vi "Nattify - Arrange FP Controls Rows.vi"(0 "sorted array of control info":T2[](array[typedef]), 1 "FP objects arrangement info":T1, 11 "error in":errorcluster) -> (15 "error out":errorcluster)   [LabVIEW 2020]
uses:
  Nattify - FP Control Info.ctl
  <vilib>/Utility/miscctls.llb/LVRectTypeDef.ctl
  Nattify - FP Objects Arrangement Info.ctl
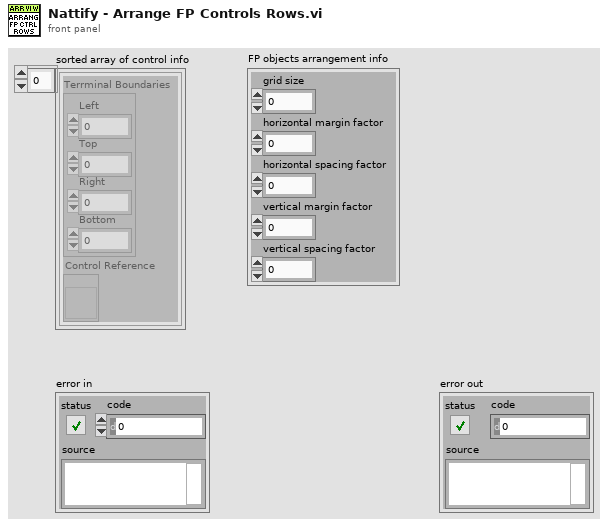
[diagram p1: front panel]
types:
  T1 = typedef "Nattify - FP Objects Arrangement Info.ctl" = cluster{"grid size":i32, "horizontal margin factor":i32, "horizontal spacing factor":i32, "vertical margin factor":i32, "vertical spacing factor":i32}
  T2 = typedef "Nattify - FP Control Info.ctl" = cluster{"Terrminal Boundaries":T3, "Control Reference":refnum<vi>}
  T3 = typedef "LVRectTypeDef.ctl" = cluster{"Left":i16, "Top":i16, "Right":i16, "Bottom":i16}
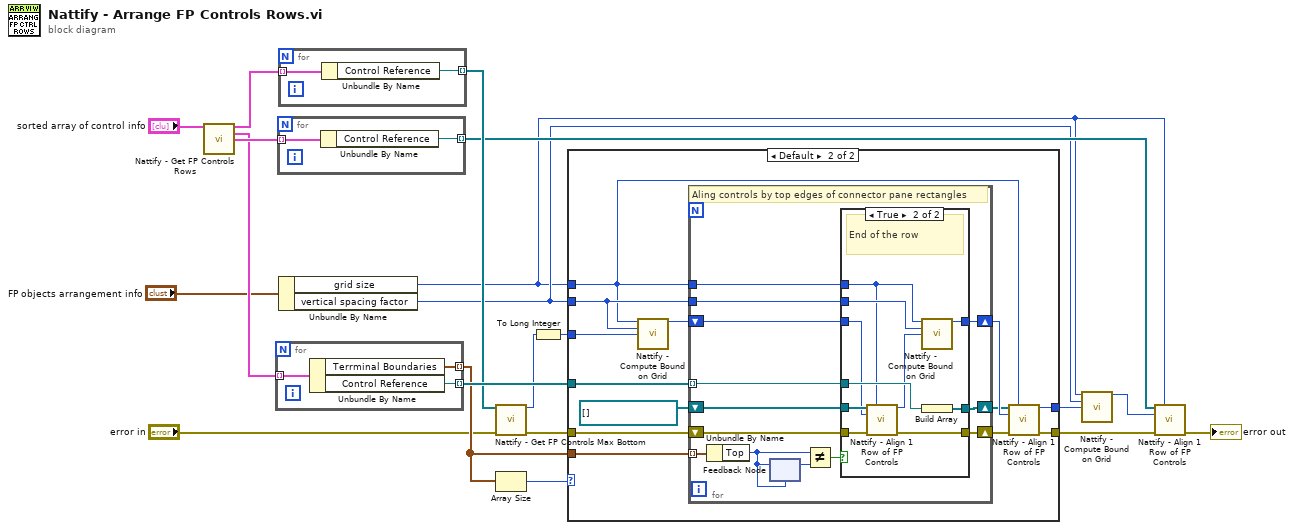
[diagram p0: block diagram]
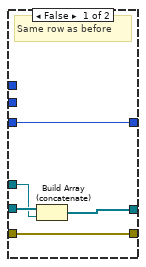
[diagram p3: hidden frame]
diagram:
  n1 = call "Nattify - Get FP Controls Rows.vi"("controls"="sorted array of control info") -> ("top row"=w18:T2[], "middle rows"=w8:T2[], "bottom row"=w13:T2[])  [unwired: 12 in]
  n2 = for {
    tunnel: w8 -> [w23] mode=indexing
    tunnel: [w22] -> w7 mode=indexing
    tunnel: [w21] -> w19 mode=indexing
    n3 = Unbundle By Name(w23) -> ("Terrminal Boundaries"=w22:T3, "Control Reference"=w21:refnum<vi>)
  }
  n4 = for {
    tunnel: w13 -> [w25] mode=indexing
    tunnel: [w24] -> w12 mode=indexing
    n5 = Unbundle By Name(w25) -> ("Control Reference"=w24:refnum<vi>)
  }
  n6 = for {
    tunnel: w18 -> [w27] mode=indexing
    tunnel: [w26] -> w17 mode=indexing
    n7 = Unbundle By Name(w27) -> ("Control Reference"=w26:refnum<vi>)
  }
  n8 = Unbundle By Name("FP objects arrangement info") -> ("grid size"=w1:i32, "vertical spacing factor"=w5:i32)
  n9 = call "Nattify - Get FP Controls Max Bottom.vi"("controls"=w17, "error in"="error in") -> ("max bottom"=w16:i16, "error out"=w15:errorcluster)  [unwired: 12 in]
  n10 = Array Size(array=w7) -> (size(s)=w4:i32)
  n11 = To Long Integer(number=w16) -> (32bit integer=w14:i32)
  n12 = case shown="Default" w4 {
    tunnel: w19 -> [_ w42]
    tunnel: w15 -> [w29 w41]
    tunnel: w14 -> [w28 w40]
    tunnel: [w29 w39] -> w11
    tunnel: w7 -> [_ w38]
    tunnel: [w28 w32] -> w6
    tunnel: w5 -> [_ w31]
    tunnel: w1 -> [_ w30]
    frame 0 {
    }
    frame Default {
      n13 = call "Nattify - Compute Bound on Grid.vi"("grid size"=w30, "grid factor"=w31, "max location (not counting spacing and grid)"=w40) -> ("computed bound on the grid"=w33:i32)  [unwired: 12 in]
      n14 = for {
        shift-right: [w54] -> w34
        shift-left: refnum<vi>[] [] -> [w53]
        shift-right: [w50] -> w37
        shift-left: w33 -> [w51]
        tunnel: w42 -> [w48] mode=indexing
        shift-right: [w43] -> w35
        shift-left: w41 -> [w49]
        tunnel: w38 -> [w47] mode=indexing
        tunnel: w31 -> [w45]
        tunnel: w30 -> [w44]
        # "Aling controls by top edges of connector pane rectangles"
        n15 = Unbundle By Name(w47) -> ("Top"=w46:i16)
        n16 = feedback-in #1(w46) -> ()
        n17 = feedback #1(w46) -> (w55:i16)
        n18 = Not Equal?(x=w46, y=w55) -> (x != y?=w52:bool)
        n19 = case shown="True" w52 {
          tunnel: [w60 w70] -> w54
          tunnel: w53 -> [w59 w67]
          tunnel: [w58 w66] -> w50
          tunnel: w51 -> [w58 w62]
          tunnel: [w57 w69] -> w43
          tunnel: w49 -> [w57 w68]
          tunnel: w48 -> [w56 w64]
          tunnel: w45 -> [_ w65]
          tunnel: w44 -> [_ w61]
          frame False {
            # "Same row as before"
            n20 = Build Array (concatenate)(w59, w56) -> (w60:refnum<vi>[])
          }
          frame True {
            # "End of the row"
            n21 = call "Nattify - Align 1 Row of FP Controls.vi"("controls"=w67, "grid size"=w61, "top bound"=w62, "error in"=w68) -> ("max bottom"=w63:i32, "error out"=w69:errorcluster)  [unwired: 10 in]
            n22 = call "Nattify - Compute Bound on Grid.vi"("grid size"=w61, "grid factor"=w65, "max location (not counting spacing and grid)"=w63) -> ("computed bound on the grid"=w66:i32)  [unwired: 12 in]
            n23 = Build Array(w64) -> (w70:refnum<vi>[])
          }
        }
      }
      n24 = call "Nattify - Align 1 Row of FP Controls.vi"("controls"=w34, "grid size"=w30, "top bound"=w37, "error in"=w35) -> ("max bottom"=w32:i32, "error out"=w39:errorcluster)  [unwired: 10 in]
    }
  }
  n25 = call "Nattify - Compute Bound on Grid.vi"("grid size"=w1, "grid factor"=w5, "max location (not counting spacing and grid)"=w6) -> ("computed bound on the grid"=w9:i32)  [unwired: 12 in]
  n26 = call "Nattify - Align 1 Row of FP Controls.vi"("controls"=w12, "grid size"=w1, "top bound"=w9, "error in"=w11) -> ("error out"=→"error out":errorcluster)  [unwired: 10 in, 1 out]
